vi "CvrtCell2Data.vi"(8 "error in":errorcluster, 9 "ge_HdrNames":T1, 10 "Item Name":string, 11 "Voltage In":refnum<class "Voltage.lvclass">) -> (0 "error out":errorcluster, 3 "Voltage Out":refnum<class "Voltage.lvclass">)   [LabVIEW 2018, in "Measurement Channels.lvlib" / "Voltage.lvclass"]
uses:
  Voltage.lvclass
  Common/Controls/HeaderNames.ctl
  SubVIs Table/Custom Ctls Table/ge_ColType.ctl
  Voltage.lvclass/Voltage.ctl
  Class Channel/Channel.lvclass
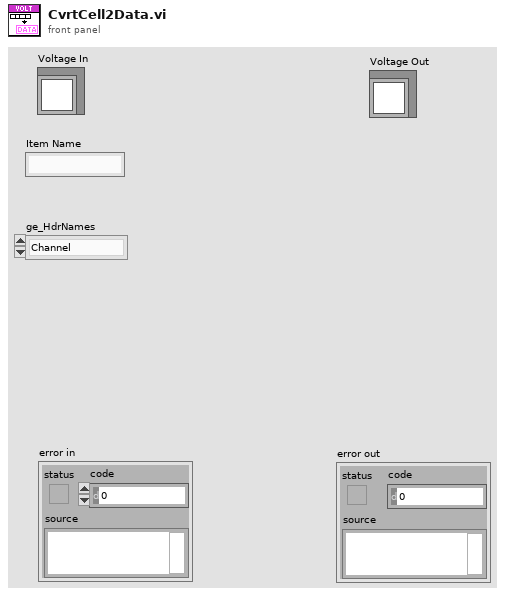
[diagram p1: front panel]
types:
  T1 = typedef "HeaderNames.ctl" = enum16{"Channel", "Device", "Spacer", "Description", "MB", "Range", "Terminal", "Coupling", "Thresh (V)", "Pulse/Rev", "Slope", "Min EU", "Min RPM", "mV/EU", "Iex", "Temp Units", "Type", "CJC Src", "CJC Val", "Ro", "Wire Cfg", "Strain Mode", "Vex", "Bridge Type", "GF", "Gauge Res", "Poisson", "Lead Res", "Init Strain", "GAF", "Scale", "Offset", "Unit (EU)", "dB?", "dB Ref", "Cal Mag", "Cal Units", "Max Temp", "Min Temp", "Max Strain", "Min Strain"}
  T2 = typedef "ge_ColType.ctl" = enum16{"Volts", "Amps", "Ohms", "TermCfg", "WireCfg", "Coup", "Slope", "Iex", "CalUnits", "ThrmUnits", "ThrmType", "CJCSrc", "BrdgType", "Strn Mode", "RTDType"}
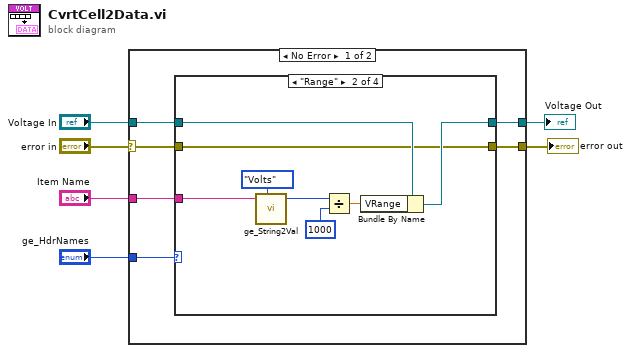
[diagram p0: block diagram]
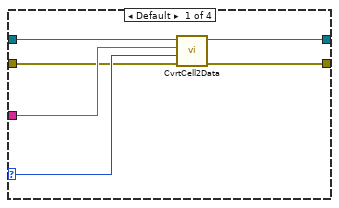
[diagram p2: hidden frame]
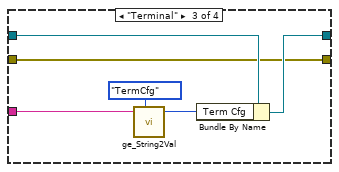
[diagram p3: hidden frame]
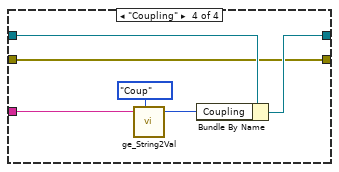
[diagram p4: hidden frame]
diagram:
  n1 = case shown="No Error" "error in" {
    selector: "error in" -> [w7 w39]
    tunnel: [w12 w40] -> w6
    tunnel: "ge_HdrNames" -> [w11 _]
    tunnel: "Item Name" -> [w10 _]
    tunnel: "Voltage In" -> [w9 w40]
    tunnel: [w8 w39] -> w2
    frame No Error {
      n2 = case shown="\"Range\"" w11 {
        selector: w11 -> [w15 _ _ _]
        tunnel: w10 -> [w16 w21 w31 w37]
        tunnel: w9 -> [w18 w26 w30 w36]
        tunnel: [w17 w25 w28 w34] -> w12
        tunnel: w7 -> [w14 w19 w27 w33]
        tunnel: [w13 w19 w27 w33] -> w8
        frame Default {
          n3 = call-parent "CvrtCell2Data.vi"("error in (no error)"=w14, "Header Names"=w15, "Item Name"=w16, "Channel in"=w18) -> ("error out"=w13:errorcluster, "Channel out"=w17:refnum<class "Voltage.lvclass">)  [unwired: 6 in]
        }
        frame "Range" {
          n4 = call "ge_String2Val.vi"("String"=w21, "ColType"=ge_ColType."Volts") -> ("Value"=w20:u16)  [unwired: 4 in, 1 out]
          n5 = Divide(x=w20, y=1000) -> (x/y=w23:dbl)
          n6 = Bundle By Name(cluster=w26, "VRange"=w23) -> (w25:refnum<class "Voltage.lvclass">)
        }
        frame "Terminal" {
          n7 = call "ge_String2Val.vi"("String"=w31, "ColType"=ge_ColType."TermCfg") -> ("Value"=w29:u16)  [unwired: 4 in, 1 out]
          n8 = Bundle By Name(cluster=w30, "Term Cfg"=w29) -> (w28:refnum<class "Voltage.lvclass">)
        }
        frame "Coupling" {
          n9 = call "ge_String2Val.vi"("String"=w37, "ColType"=ge_ColType."Coup") -> ("Value"=w35:u16)  [unwired: 4 in, 1 out]
          n10 = Bundle By Name(cluster=w36, "Coupling"=w35) -> (w34:refnum<class "Voltage.lvclass">)
        }
      }
    }
    frame Error {
    }
  }
  "Voltage Out" <- w6
  "error out" <- w2
